vi "Hallway to Room.vi"(8 "error in (no error)":errorcluster, 10 "LRU Cache in":refnum<class "LRU Cache.lvclass">, 11 "State in":refnum<class "State.lvclass">) -> (0 "error out":errorcluster, 1 "Moved?":bool, 2 "LRU Cache out":refnum<class "LRU Cache.lvclass">, 3 "State out":refnum<class "State.lvclass">)   [LabVIEW 2019, in "23.lvlib" / "State.lvclass"]
uses:
  State.lvclass
  C:/Users/craig.walker/Documents/GitHub/lv2019-LRU-Cache/LRU Node/LRU Node.lvclass
  lv2019-LRU-Cache/LRU Cache/LRU Cache.lvclass
  lv2019-LRU-Cache/LRU Node/LRU Node.lvclass/LRU Node.ctl
  State Key/State Key.lvclass/State Key.ctl
  State Value/State Value.lvclass/State Value.ctl
  lv2019-LRU-Cache/LRU Node/Read Key.vi
  Between.vi
  lv2019-LRU-Cache/LRU Node/Write Key.vi
  lv2019-LRU-Cache/LRU Node/Write Value.vi
  lv2019-LRU-Cache/LRU Node/Read Value.vi
  State Key/State Key.lvclass
  State Value/State Value.lvclass
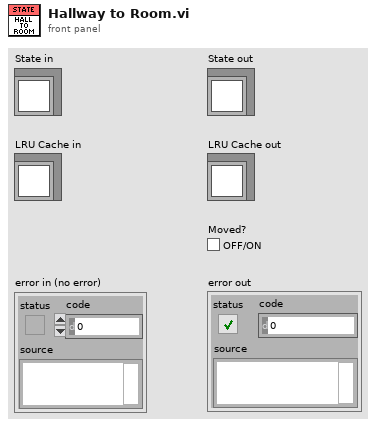
[diagram p1: front panel]
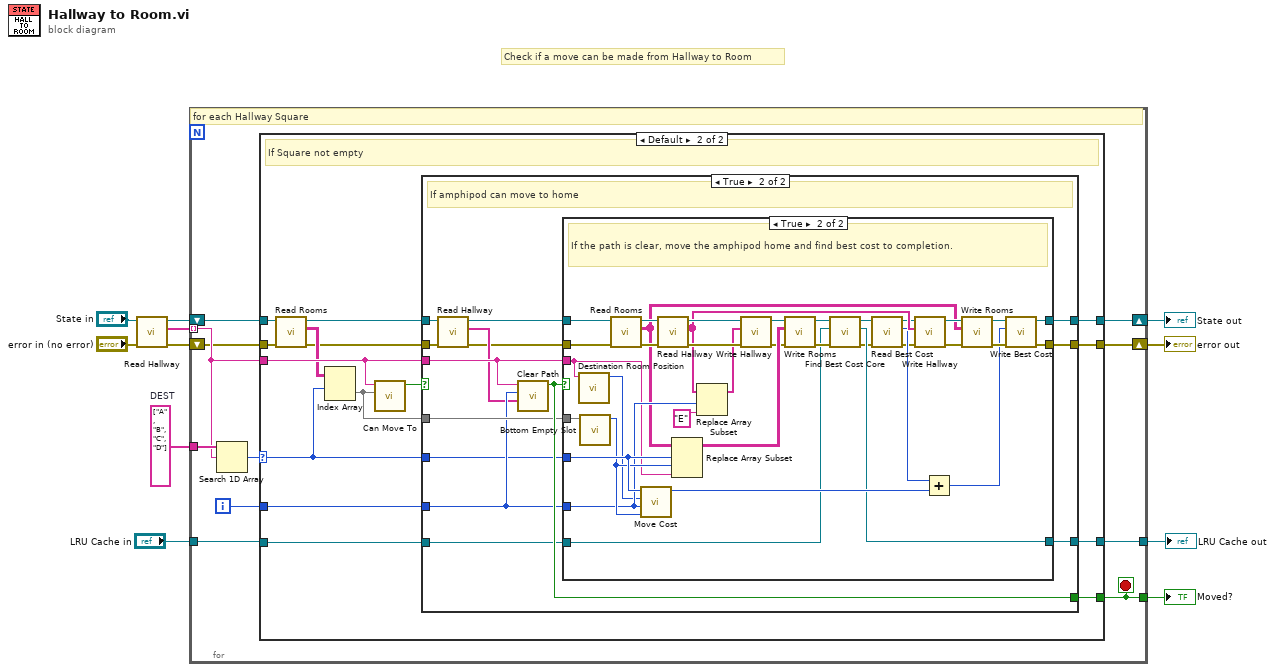
[diagram p0: block diagram]
diagram:
  w6 = string[] ["A", "B", "C", "D"]  # DEST
  # "Check if a move can be made from Hallway to Room"
  n1 = call "Read Hallway.vi"("error in (no error)"="error in (no error)", "State in"="State in") -> ("error out"=w4:errorcluster, "Hallway"=w7:string[], "State out"=w5:refnum<class "State.lvclass">)  [unwired: 7 in]
  n2 = for {
    tunnel: w7 -> [w18] mode=indexing
    tunnel: w6 -> [w22]
    tunnel: [w20] -> w11
    shift-right: [w13] -> w1
    shift-left: w4 -> [w14]
    shift-right: [w12] -> w3
    shift-left: w5 -> [w15]
    tunnel: "LRU Cache in" -> [w17]
    tunnel: [w16] -> w9
    i -> [w21]
    stop <- w20 stop-if-true
    # "for each Hallway Square"
    n3 = Search 1D Array(1D array=w22, element=w18) -> (index of element=w19:i32)  [unwired: 1 in]
    n4 = case shown="Default" w19 {
      selector: w19 -> [_ w35]
      tunnel: w21 -> [_ w40]
      tunnel: w18 -> [_ w39]
      tunnel: [_ w37] -> w20
      tunnel: w17 -> [w25 w34]
      tunnel: [w25 w33] -> w16
      tunnel: w15 -> [w24 w32]
      tunnel: w14 -> [w23 w29]
      tunnel: [w23 w27] -> w13
      tunnel: [w24 w26] -> w12
      frame -1 {
        # "if position empty try next position"
      }
      frame Default {
        # "If Square not empty"
        n5 = call "Read Rooms.vi"("error in (no error)"=w29, "State in"=w32) -> ("error out"=w28:errorcluster, "Rooms"=w30:string[][], "State out"=w31:refnum<class "State.lvclass">)  [unwired: 7 in]
        n6 = Index Array(array=w30, index (row)=w35) -> (element=w36:string[])  [unwired: 1 in]
        n7 = call "Can Move To.vi"("Room"=w36, "Amphipod Type"=w39) -> ("Can Move To?"=w38:bool)  [unwired: 9 in]
        n8 = case shown="True" w38 {
          tunnel: w40 -> [_ w54]
          tunnel: w39 -> [_ w57]
          tunnel: [_ w56] -> w37
          tunnel: w36 -> [_ w55]
          tunnel: w35 -> [_ w53]
          tunnel: w34 -> [w43 w52]
          tunnel: [w43 w51] -> w33
          tunnel: w31 -> [w42 w49]
          tunnel: w28 -> [w41 w47]
          tunnel: [w41 w45] -> w27
          tunnel: [w42 w44] -> w26
          frame False {
            # "If amphipod in position can't move home, try next position"
          }
          frame True {
            # "If amphipod can move to home"
            n9 = call "Read Hallway.vi"("error in (no error)"=w47, "State in"=w49) -> ("error out"=w46:errorcluster, "Hallway"=w50:string[], "State out"=w48:refnum<class "State.lvclass">)  [unwired: 7 in]
            n10 = call "Clear Path.vi"("Hallway"=w50, "Hallway Position"=w54, "Room"=w57) -> ("Clear Path?"=w56:bool)  [unwired: 8 in]
            n11 = case shown="True" w56 {
              tunnel: w57 -> [_ w89]
              tunnel: w55 -> [_ w96]
              tunnel: w54 -> [_ w91]
              tunnel: w53 -> [_ w93]
              tunnel: w52 -> [w60 w77]
              tunnel: [w60 w76] -> w51
              tunnel: w48 -> [w59 w85]
              tunnel: w46 -> [w58 w83]
              tunnel: [w58 w67] -> w45
              tunnel: [w59 w69] -> w44
              frame False {
                # "if path is not clear, try next position"
              }
              frame True {
                # "If the path is clear, move the amphipod home and find best cost to completion."
                n12 = call "Destination Room Position.vi"("Amphipod Type"=w89) -> ("Destination Room Position"=w90:i32)  [unwired: 10 in]
                n13 = call "Bottom Empty Slot.vi"("Room"=w96) -> ("Slot"=w92:i32)  [unwired: 10 in]
                n14 = call "Read Rooms.vi"("error in (no error)"=w83, "State in"=w85) -> ("error out"=w82:errorcluster, "Rooms"=w71:string[][], "State out"=w84:refnum<class "State.lvclass">)  [unwired: 7 in]
                n15 = call "Move Cost.vi"("Room Slot"=w92, "Destination Position"=w91, "Source Position"=w90, "Amphipod Type Index"=w93) -> ("Move Cost"=w95:u64)  [unwired: 7 in]
                n16 = call "Read Hallway.vi"("error in (no error)"=w82, "State in"=w84) -> ("error out"=w81:errorcluster, "Hallway"=w74:string[], "State out"=w78:refnum<class "State.lvclass">)  [unwired: 7 in]
                n17 = Replace Array Subset(array=w71, new element=w89, index (row)=w93, index (col)=w92) -> (w87:string[][])
                n18 = Replace Array Subset(array=w74, new element="E" ("y"), index=w91) -> (w75:string[])
                n19 = call "Write Hallway.vi"("error in (no error)"=w81, "Hallway"=w75, "State in"=w78) -> ("error out"=w80:errorcluster, "State out"=w88:refnum<class "State.lvclass">)  [unwired: 7 in]
                n20 = call "Write Rooms.vi"("error in (no error)"=w80, "Rooms"=w87, "State in"=w88) -> ("error out"=w79:errorcluster, "State out"=w86:refnum<class "State.lvclass">)  [unwired: 7 in]
                n21 = call "Find Best Cost Core.vi"("error in (no error)"=w79, "LRU Cache in"=w77, "State in"=w86) -> ("error out"=w63:errorcluster, "LRU Cache out"=w76:refnum<class "LRU Cache.lvclass">, "State out"=w65:refnum<class "State.lvclass">)  [unwired: 6 in]
                n22 = call "Read Best Cost.vi"("error in (no error)"=w63, "State in"=w65) -> ("error out"=w61:errorcluster, "Best Cost"=w64:u64, "State out"=w62:refnum<class "State.lvclass">)  [unwired: 7 in]
                n23 = call "Write Hallway.vi"("error in (no error)"=w61, "Hallway"=w74, "State in"=w62) -> ("error out"=w73:errorcluster, "State out"=w72:refnum<class "State.lvclass">)  [unwired: 7 in]
                n24 = Add(x=w64, y=w95) -> (x+y=w66:u64)
                n25 = call "Write Rooms.vi"("error in (no error)"=w73, "Rooms"=w71, "State in"=w72) -> ("error out"=w68:errorcluster, "State out"=w70:refnum<class "State.lvclass">)  [unwired: 7 in]
                n26 = call "Write Best Cost.vi"("error in (no error)"=w68, "Best Cost"=w66, "State in"=w70) -> ("error out"=w67:errorcluster, "State out"=w69:refnum<class "State.lvclass">)  [unwired: 7 in]
              }
            }
          }
        }
      }
    }
  }
  "Moved?" <- w11
  "State out" <- w3
  "LRU Cache out" <- w9
  "error out" <- w1
